vi "Lim_InitPicture.vi"(8 "error in (no error)":errorcluster, 10 "LIMATTRIBUTES":T2, 11 "hFile in":T1) -> (0 "error out":errorcluster, 1 "LIMSIZE":u32, 2 "LIMPICTURE":T3, 3 "hFile out":T1)   [LabVIEW 2014, in "ND2_Reader_32.lvlib"]
doc: "This routine creates data space that is used when reading a frame out of the file."
uses:
  ND2_Reader_32.lvlib
  controls/cluster_LIMPICTURE.ctl
  controls/cluster_LIMATTRIBUTES.ctl
  controls/numeric_LIMFILEHANDLE.ctl
  nd2 reader/SDK/bin/x86/v6_w32_nd2ReadSDK.dll
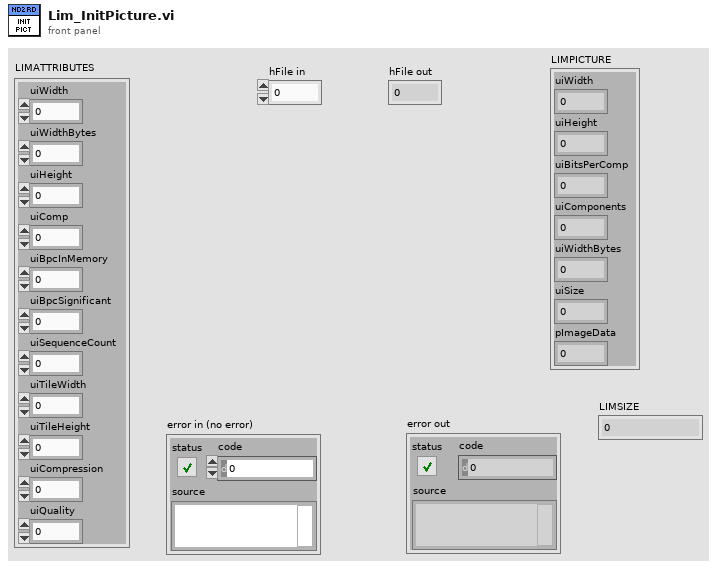
[diagram p1: front panel]
types:
  T1 = typedef "numeric_LIMFILEHANDLE.ctl" = i32
  T2 = typedef "cluster_LIMATTRIBUTES.ctl" = cluster{"uiWidth":u32, "uiWidthBytes":u32, "uiHeight":u32, "uiComp":u32, "uiBpcInMemory":u32, "uiBpcSignificant":u32, "uiSequenceCount":u32, "uiTileWidth":u32, "uiTileHeight":u32, "uiCompression":u32, "uiQuality":u16}
  T3 = typedef "cluster_LIMPICTURE.ctl" = cluster{"uiWidth":u32, "uiHeight":u32, "uiBitsPerComp":u32, "uiComponents":u32, "uiWidthBytes":u32, "uiSize":u32, "pImageData":u32}
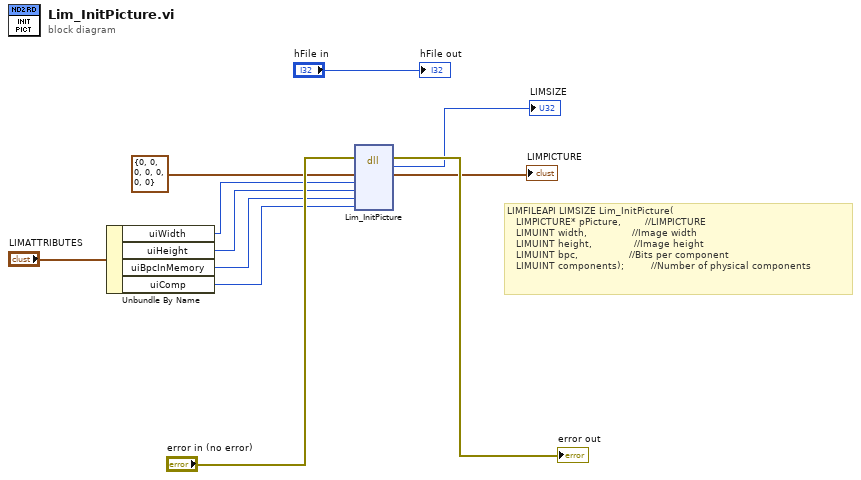
[diagram p0: block diagram]
diagram:
  # "LIMFILEAPI LIMSIZE Lim_InitPicture(\n   LIMPICTURE* pPicture,        //LIMPICTURE\n   LIMUINT width,               //Image width\n   LIMUINT height,              //Image height\n   LIMUINT bpc,                 //Bits per component\n   LIMUINT components);         //Number of physical components"
  n1 = Unbundle By Name("LIMATTRIBUTES") -> ("uiWidth"=w6:u32, "uiHeight"=w5:u32, "uiBpcInMemory"=w3:u32, "uiComp"=w2:u32)
  n2 = dll-call lib="C:/Users/VirtualUser/Desktop/EPA-Vision/EPA Image Source LV2014 2.0.0 2016-02-23/ND2_Reader_32bit/nd2 reader/SDK/bin/x86/v6_w32_nd2ReadSDK.dll" fn="Lim_InitPicture"(error in="error in (no error)", "pPicture"=T3 {"uiWidth"=0, "uiHeight"=0, "uiBitsPerComp"=0, "uiComponents"=0, "uiWidthBytes"=0, "uiSize"=0, "pImageData"=0} ("LIMPICTURE"), "width"=w6, "height"=w5, "bpc"=w3, "components"=w2) -> (error out=→"error out":errorcluster, "LIMSIZE"=→"LIMSIZE":u32, "pPicture"=→"LIMPICTURE":T3)  [unwired: 2 in, 5 out]
  "hFile out" <- "hFile in"
